vi "Focus Set Home.vi"(8 "error in (no error)":errorcluster, 10 "Motor (0:n-1)":i32, 11 "NewFocus in":refnum<class "NewFocus.lvclass">) -> (0 "error out":errorcluster, 3 "NewFocus out":refnum<class "NewFocus.lvclass">)   [LabVIEW 2021, in "NewFocus.lvclass"]
uses:
  NewFocus.lvclass
  C:/Development/prime/Prime-RIMAS/Focus/Focus Class/Focus Class.lvclass
  NewFocus.lvclass/NewFocus.ctl
  Focus Class/Focus Class.lvclass
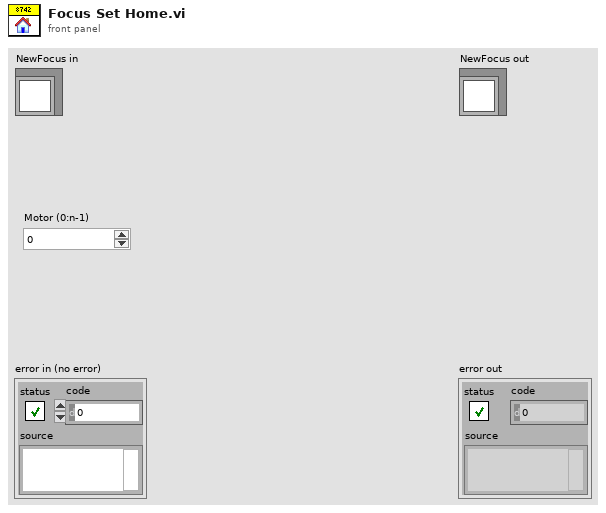
[diagram p1: front panel]
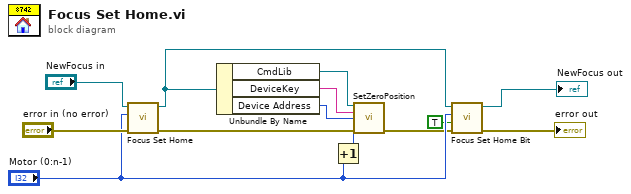
[diagram p0: block diagram]
diagram:
  n1 = call-parent "Focus Set Home.vi"("error in (no error)"="error in (no error)", "Motor (0:n-1)"="Motor (0:n-1)", "Focus Class in"="NewFocus in") -> ("error out"=w8:errorcluster, "Focus Class out"=w7:refnum<class "NewFocus.lvclass">)  [unwired: 7 in]
  n2 = Unbundle By Name(w7) -> ("CmdLib"=w11:refnum<k24>, "DeviceKey"=w10:string, "Device Address"=w9:i32)
  n3 = Increment(x="Motor (0:n-1)") -> (x+1=w1:i32)
  n4 = call "SetZeroPosition.vi"("CmdLib In"=w11, "DeviceKey In"=w10, "Device Address In"=w9, "Motor"=w1, "error in (no error)"=w8) -> ("error out"=w5:errorcluster)  [unwired: 7 in, 3 out]
  n5 = call "Focus Set Home Bit.vi"("error in (no error)"=w5, "Homed?"=TRUE, "Motor (0:n-1)"="Motor (0:n-1)", "Focus Class in"=w7) -> ("error out"=→"error out":errorcluster, "Focus Class out"=→"NewFocus out":refnum<class "NewFocus.lvclass">)  [unwired: 6 in]
